vi "setData.vi"(8 "error in (no error)":errorcluster, 10 "Data":T1={"Timestamps ms"=[0.0, 0.005, 0.009, 0.012], "DataPerChannel"=[]} {"Timestamps ms" format="%.3f"}, 11 "DigitalOutput.lvclass in":refnum<class "DigitalOutput.lvclass">) -> (0 "error out":errorcluster, 3 "DigitalOutput.lvclass out":refnum<class "DigitalOutput.lvclass">)   [LabVIEW 2011, in "Hardware.lvlib" / "Channels.lvlib" / "DigitalOutput.lvclass"]
uses:
  DigitalOutput.lvclass
  DigitalOutput.lvclass/DigitalOutput.ctl
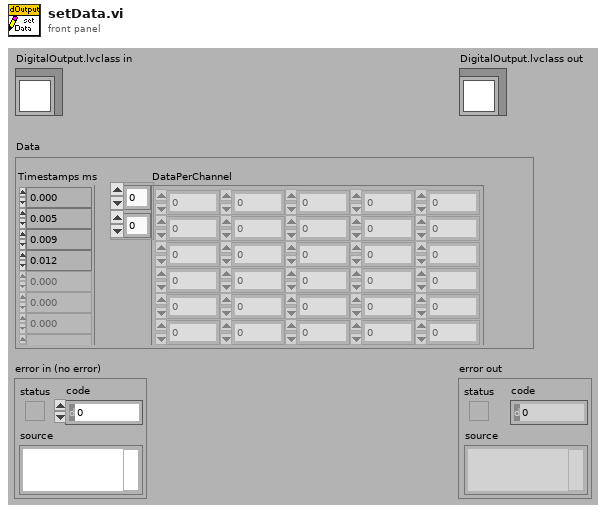
[diagram p1: front panel]
types:
  T1 = cluster{"Timestamps ms":dbl[], "DataPerChannel":dbl[][]}
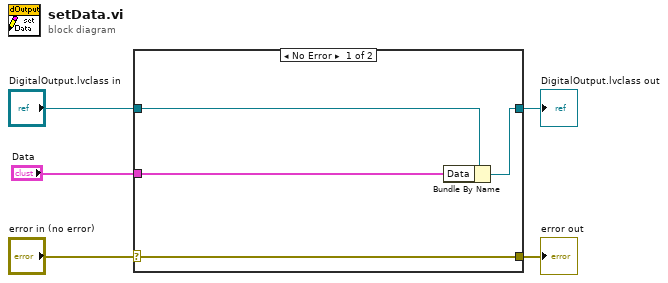
[diagram p0: block diagram]
diagram:
  n1 = case shown="No Error" "error in (no error)" {
    selector: "error in (no error)" -> [w9 w10]
    tunnel: [w9 w10] -> w4
    tunnel: [w7 w11] -> w2
    tunnel: "DigitalOutput.lvclass in" -> [w8 w11]
    tunnel: "Data" -> [w6 _]
    frame No Error {
      n2 = Bundle By Name(cluster=w8, "Data"=w6) -> (w7:refnum<class "DigitalOutput.lvclass">)
    }
    frame Error {
    }
  }
  "error out" <- w4
  "DigitalOutput.lvclass out" <- w2
